vi "USBL_UA TRACKER for boat_rev2.vi"() -> ()   [LabVIEW 2017]
uses:
  <vilib>/Analysis/2dsp.llb/Decimate (single shot, DBL).vi
  <vilib>/DAQmx/read.llb/DAQmx Read (Analog 1D Wfm NChan NSamp).vi
  <vilib>/Analysis/3filter.llb/FIR Filter (DBL).vi
  <vilib>/DAQmx/create/channels.llb/DAQmx Create Channel (AI-Voltage-Basic).vi
  <vilib>/DAQmx/configure/timing.llb/DAQmx Timing (Sample Clock).vi
  <vilib>/DAQmx/miscellaneous.llb/DAQmx Fill In Error Info.vi
  <vilib>/DAQmx/create/channels.llb/DAQmx Create Channel (CO-Pulse Generation-Frequency).vi
  <vilib>/DAQmx/configure/timing.llb/DAQmx Timing (Implicit).vi
  <vilib>/Analysis/NI_AALBase.lvlib
  <vilib>/Analysis/NI_AALPro.lvlib
  <vilib>/Analysis/NI_AAL_SigProc.lvlib
  <resource>/objmgr/daqmx.rc
panel:
  out "숫자형 8":dbl=5.0
  out "Target code":dbl[](array[numeric])
  out "ThresholdMargin":dbl=10.0
  out "MovingAvrParm":dbl[](array[numeric])
  out "Coefficient_bit1":dbl[](array[numeric])
  out "Coefficient_bit0":dbl[](array[numeric])
  out "Decimation rate":i32=12
  out "Carrier signal":dbl[](array[numeric])
  out "숫자형 7":dbl=7.0
  out "숫자형 6":dbl=7.0
  out "숫자형 5":dbl=7.0
  in  "Number of pulse":i32=1000
  in  "Output terminal":tag="/Dev1/PFI12"
  in  "Frequency(Hz)":dbl=1.0 format="%.6f"
  in  "Cycle share":dbl=0.5 format="%.6f"
  in  "Counter":tag="Dev1/ctr0"
  out "Detect":bool
  in  "User number":i32=12
  out "숫자형 4":dbl=5.0
  out "숫자형 3":dbl=7.0
  out "숫자형 2":dbl=7.0
  out "숫자형":dbl=7.0
  in  "Start frequency(Hz)":dbl format="%#_6p"
  in  "Stop frequency(Hz)":dbl=4000.0 format="%#_6p"
  in  "Symbol length(sec)":dbl=0.128 format="%#_6p"
  in  "Number of sample":i32=38400
  in  "Sampling freuqncy(Hz)":dbl=192000.0 format="%#_6p"
  in  "Physical channel":tag="Dev4/ai0:7" caption="Physical Channel"
  in  "Device":tag="Dev4"
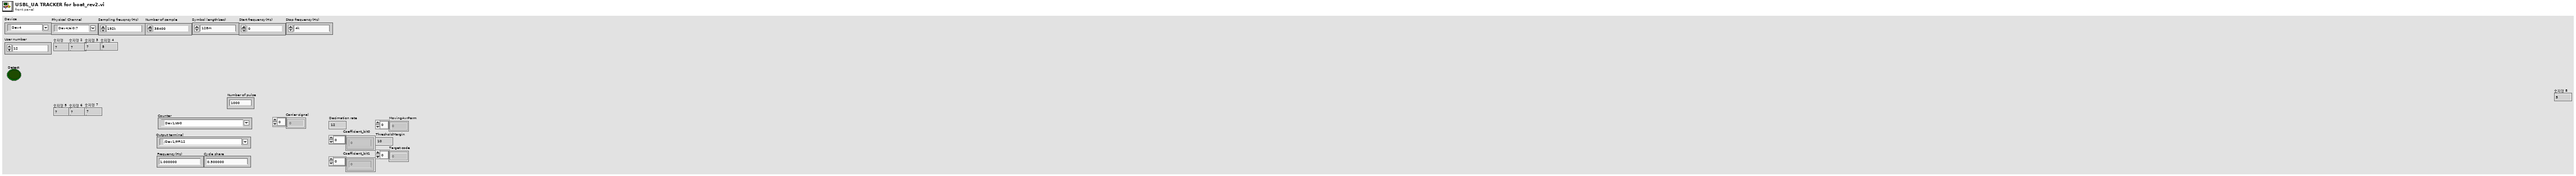
[diagram p1: front panel]
diagram:
  n1 = flat-sequence {
    tunnel: ["Number of sample"] -> w12
    tunnel: [w39] -> w11
    tunnel: ["Sampling freuqncy(Hz)"] -> w10
    tunnel: ["Physical channel"] -> w9
    tunnel: ["Device"] -> w8
    tunnel: [w35] -> w7
    tunnel: [w31] -> w6
    tunnel: [w30] -> w5
    tunnel: [w25] -> w4
    tunnel: [w21] -> w3
    tunnel: [w20] -> w2
    tunnel: [w13] -> w1
    tunnel: w12 -> [w59]
    tunnel: w11 -> [w58]
    tunnel: w10 -> [w57]
    tunnel: w9 -> [w56]
    tunnel: w8 -> [w55]
    tunnel: w7 -> [w54]
    tunnel: w6 -> [w53]
    tunnel: w5 -> [w52]
    tunnel: w4 -> [w49]
    tunnel: w3 -> [w47]
    tunnel: w2 -> [w46]
    tunnel: w1 -> [w43]
    frame #0 {
      w20 = 10.0 ("값")
      w22 = 160 ("차원 크기")
      w35 = 12 ("Divide by")
      w39 = 10123 items=["유한 샘플"=10178, "연속 샘플"=10123, "하드웨어 타이밍에 의한 단일 포인트"=12522] ("sample mode")
      # "Signal gen. (Counter)"
      # "Target code"
      # "EOF"
      # "SOF"
      # "Processing parameter"
      # "Freqeuncy 2"
      # "Freqeuncy 1"
      # "Symbol length"
      # "Moving average window size"
      # "Threshold Margin"
      # "DAQ device setting"
      # "Device"
      # "Physical channel"
      # "Sampling frequency"
      # "Sample mode"
      # "Number of samples per channel"
      n2 = To Double Precision Float(number=w35) -> (double precision float=w41:dbl)
      n3 = To Double Precision Float(number=w22) -> (double precision float=w24:dbl)
      n4 = Divide(x="Sampling freuqncy(Hz)", y=w41) -> (x/y=w29:dbl)
      n5 = Format Into String(format string="%04b" ("포맷 문자열"), "User number") -> (resulting string=w17:string)  [unwired: 2 in, 1 out]
      n6 = Reciprocal(x=w24) -> (1/x=w23:dbl)
      n7 = call "CodeConvert(SubVI).vi"("Code"=w17) -> ("Code_array"=w15:dbl[])
      n8 = Divide(x=30000.0, y="Sampling freuqncy(Hz)") -> (x/y=w33:dbl)
      n9 = Initialize Array(w23, w22) -> (w21:dbl[])
      "MovingAvrParm" <- w21
      n10 = call "ChirpSourceGen(SubVI).vi"("Frequency2(Hz)"="Stop frequency(Hz)", "Frequency1(Hz)"="Start frequency(Hz)", "Pulse length(sec)"="Symbol length(sec)", "Fs(Hz)"=w29) -> ("M.F. Tap(F2-1)"=w25:dbl[], "M.F. Tap(F1-2)"=w31:dbl[])  [unwired: 1 out]
      "Coefficient_bit0" <- w31
      "Coefficient_bit1" <- w25
      n11 = Insert Into Array(array=dbl[] [0.0, 1.0], new element #1=w15, new element #2=dbl[] [1.0, 0.0]) -> (w13:dbl[])  [unwired: 1 in]
      "Target code" <- w13
      n12 = call <vilib>:"Sine Wave.vi"("samples"="Number of sample", "amplitude"=5.0, "frequency"=w33) -> ("sine wave"=w30:dbl[])  [unwired: 2 in, 2 out]
      "Carrier signal" <- w30
      "Decimation rate" <- w35
      "ThresholdMargin" <- w20
    }
    frame #1 {
      n13 = flat-sequence {
        tunnel: w55 -> [w78]
        tunnel: [w79] -> w66
        tunnel: w56 -> [w77]
        tunnel: [w77] -> w65
        tunnel: w57 -> [w75]
        tunnel: [w75] -> w64
        tunnel: w59 -> [w74]
        tunnel: [w74] -> w63
        tunnel: w58 -> [w76]
        tunnel: [w76] -> w62
        tunnel: [w72] -> w61
        tunnel: [w73] -> w60
        tunnel: w54 -> [w73]
        tunnel: w53 -> [w72]
        tunnel: w52 -> [w71]
        tunnel: [w71] -> w51
        tunnel: [w70] -> w50
        tunnel: w49 -> [w70]
        tunnel: [w69] -> w48
        tunnel: w47 -> [w69]
        tunnel: w46 -> [w68]
        tunnel: [w68] -> w45
        tunnel: [w67] -> w44
        tunnel: w43 -> [w67]
        tunnel: w66 -> [w123]
        tunnel: w65 -> [w122]
        tunnel: w64 -> [w121]
        tunnel: w63 -> [w119]
        tunnel: w62 -> [w120]
        tunnel: w61 -> [w108]
        tunnel: w60 -> [w96]
        tunnel: w51 -> [w97]
        tunnel: w50 -> [w81]
        tunnel: w48 -> [w88]
        tunnel: w45 -> [w87]
        tunnel: w44 -> [w82]
        tunnel: [w407] -> w42
        tunnel: w42 -> [w500]
        frame #0 {
          n14 = call <vilib>:"DAQmx Reset Device.vi"("device in"=w78) -> ("error out"=w79:errorcluster)  [unwired: 1 in, 13 out]
        }
        frame #1 {
          w94 = "Proc1" ("이름(이름없음)")
          w95 = "Proc0" ("이름(이름없음)")
          w93 = dbl[][] []
          w109 = "SIG0" ("이름(이름없음)")
          w116 = waveform(dbl) {"t0"=timestamp(0 s since 1904-01-01), "dt"=1.0, "Y"=[]} ("Waveform")
          w99 = "SIG1" ("이름(이름없음)")
          # "Target code"
          # "[Post processing]  1. Queue get : Proc0, Proc1 / 2. Threshold estimation with moving average / 3. Peak and valley detection / 4. Demodulation"
          # "[Signal processing]\n1. Queue get : SIG0\n2. Data type converting : Waveform (DBL) --> Array (DBL)\n3. DDC (Digital to Digital Convering)\n  - DSB modulation : Multiply carrier signal (30kHz)\n  - Decimate : 192kHz sample rate --> 16kHz sample rate\n4. Cross-correlation with down-chirp (4k ~ 0Hz)\n5. Envelope detection (Hilbert transform) & square\n6. Queue put : Proc1"
          # "[Signal processing]\n1. Queue get : SIG0\n2. Data type converting : Waveform (DBL) --> Array (DBL)\n3. DDC (Digital to Digital Convering)\n  - DSB modulation : Multiply carrier signal (30kHz)\n  - Decimate : 192kHz sample rate --> 16kHz sample rate\n4. Cross-correlation with up-chirp (0 ~ 4kHz)\n5. Envelope detection (Hilbert transform) & square\n6. Queue put : Proc0"
          # "[Data Acquistion (ADC)]\n1. Device reset\n2. Creat channel\n3, Set sample clock\n  - Sampling frequency : 192kHz\n  - Number of sample (Chunk size) : 38400\n4. Start task\n5. Data read\n6. Queue put : SIG0, SIG1\n  - Queue data type : Waveform (DBL)"
          # "Moving average prameter based on FIR filter calculation"
          # "Coefficient for bit 1 : Down-chirp"
          # "Coefficient for bit 0 : Up-chirp"
          # "Decimation rate"
          # "Carrier signal"
          n15 = call-poly <vilib>:"DAQmx Create Virtual Channel.vi"("physical channels"=w122, "error in"=w123) -> ("task out"=w125:refnum<k21>, "error out"=w124:errorcluster)  [unwired: 7 in, 5 out]
          n16 = call-poly <vilib>:"DAQmx Timing.vi"("task/channels in"=w125, "sample mode"=w120, "samples per channel"=w119, "rate"=w121, "error in"=w124) -> ("task out"=w126:refnum<k21>, "error out"=w127:errorcluster)  [unwired: 2 in, 7 out]
          n17 = call <vilib>:"DAQmx Start Task.vi"("task/channels in"=w126, "error in"=w127) -> ("task out"=w128:refnum<k21>, "error out"=w129:errorcluster)  [unwired: 12 in]
          n18 = Build Array(w116, w116, w116, w116, w116, w116, w116, w116) -> (w98:waveform(dbl)[])
          n19 = Obtain Queue(name (unnamed)=w99, element data type=w98) -> (queue out=w118:refnum<queue>, error out=w117:errorcluster)  [unwired: 3 in, 1 out]
          n20 = Obtain Queue(name (unnamed)=w109, element data type=w98) -> (queue out=w115:refnum<queue>, error out=w114:errorcluster)  [unwired: 3 in, 1 out]
          n21 = while {
            tunnel: w128 -> [w406]
            tunnel: w129 -> [w405]
            tunnel: [w404] -> w132
            tunnel: [w403] -> w133
            tunnel: w119 -> [w402]
            tunnel: w118 -> [w401]
            tunnel: w117 -> [w400]
            tunnel: w115 -> [w399]
            tunnel: w114 -> [w398]
            i -> [w396]
            stop <- w395 stop-if-true
            n22 = call-poly <vilib>:"DAQmx Read.vi"("task/channels in"=w406, "number of samples per channel"=w402, "error in"=w405) -> ("task out"=w404:refnum<k21>, "data"=w397:waveform(dbl)[], "error out"=w403:errorcluster)  [unwired: 10 out]
            n23 = Enqueue Element(queue=w399, element=w397, error in (no error)=w398) -> ()  [unwired: 1 in, 3 out]
            n24 = Enqueue Element(queue=w401, element=w397, error in (no error)=w400) -> ()  [unwired: 1 in, 3 out]
            n25 = local read "Detect"() -> (w395:bool)
            "숫자형" <- w396
          }
          n26 = call <vilib>:"DAQmx Stop Task.vi"("task/channels in"=w132, "error in"=w133) -> ("task out"=w131:refnum<k21>, "error out"=w130:errorcluster)  [unwired: 12 out]
          n27 = call <vilib>:"DAQmx Clear Task.vi"("task in"=w131, "error in"=w130) -> ()  [unwired: 14 out]
          n28 = Obtain Queue(name (unnamed)=w95, element data type=w93) -> (queue out=w113:refnum<queue>, error out=w112:errorcluster)  [unwired: 3 in, 1 out]
          n29 = Obtain Queue(name (unnamed)=w109, element data type=w98) -> (queue out=w111:refnum<queue>, error out=w110:errorcluster)  [unwired: 3 in, 1 out]
          n30 = while {
            tunnel: w111 -> [w394]
            tunnel: w110 -> [w393]
            tunnel: w113 -> [w392]
            tunnel: w112 -> [w391]
            tunnel: [w390] -> w107
            tunnel: [w389] -> w106
            tunnel: w97 -> [w329]
            tunnel: w96 -> [w328]
            tunnel: w108 -> [w327]
            i -> [w325]
            stop <- w324 stop-if-true
            w339 = TRUE ("averaging")
            w388 = TRUE ("init/cont (init:F)")
            n31 = Dequeue Element(queue=w394, error in (no error)=w393) -> (queue out=w390:refnum<queue>, element=w330:waveform(dbl)[], error out=w389:errorcluster)  [unwired: 2 out]
            n32 = Index Array(array=w330) -> (element #1=w387:waveform(dbl), element #2=w386:waveform(dbl), element #3=w385:waveform(dbl), element #4=w384:waveform(dbl), element #5=w383:waveform(dbl), element #6=w382:waveform(dbl), element #7=w381:waveform(dbl), element #8=w380:waveform(dbl))  [unwired: 8 in]
            n33 = Unbundle By Name(w387) -> ("Y"=w379:dbl[])
            n34 = Unbundle By Name(w386) -> ("Y"=w378:dbl[])
            n35 = Unbundle By Name(w385) -> ("Y"=w377:dbl[])
            n36 = Unbundle By Name(w384) -> ("Y"=w376:dbl[])
            n37 = Unbundle By Name(w383) -> ("Y"=w375:dbl[])
            n38 = Unbundle By Name(w382) -> ("Y"=w374:dbl[])
            n39 = Unbundle By Name(w381) -> ("Y"=w373:dbl[])
            n40 = Unbundle By Name(w380) -> ("Y"=w372:dbl[])
            n41 = Multiply(x=w379, y=w329) -> (x*y=w354:dbl[])
            n42 = Multiply(x=w378, y=w329) -> (x*y=w353:dbl[])
            n43 = Multiply(x=w377, y=w329) -> (x*y=w352:dbl[])
            n44 = Multiply(x=w376, y=w329) -> (x*y=w351:dbl[])
            n45 = Multiply(x=w375, y=w329) -> (x*y=w350:dbl[])
            n46 = Multiply(x=w374, y=w329) -> (x*y=w349:dbl[])
            n47 = Multiply(x=w373, y=w329) -> (x*y=w348:dbl[])
            n48 = Multiply(x=w372, y=w329) -> (x*y=w347:dbl[])
            n49 = call-poly <vilib>:"Decimate (single shot).vi"("averaging"=w339, "decimating factor"=w328, "X"=w349) -> ("Decimated Array"=w342:dbl[])  [unwired: 7 in, 1 out]
            n50 = call-poly <vilib>:"Decimate (single shot).vi"("averaging"=w339, "decimating factor"=w328, "X"=w347) -> ("Decimated Array"=w340:dbl[])  [unwired: 7 in, 1 out]
            n51 = call-poly <vilib>:"Decimate (single shot).vi"("averaging"=w339, "decimating factor"=w328, "X"=w353) -> ("Decimated Array"=w346:dbl[])  [unwired: 7 in, 1 out]
            n52 = call-poly <vilib>:"Decimate (single shot).vi"("averaging"=w339, "decimating factor"=w328, "X"=w351) -> ("Decimated Array"=w344:dbl[])  [unwired: 7 in, 1 out]
            n53 = call-poly <vilib>:"Decimate (single shot).vi"("averaging"=w339, "decimating factor"=w328, "X"=w350) -> ("Decimated Array"=w343:dbl[])  [unwired: 7 in, 1 out]
            n54 = call-poly <vilib>:"Decimate (single shot).vi"("averaging"=w339, "decimating factor"=w328, "X"=w348) -> ("Decimated Array"=w341:dbl[])  [unwired: 7 in, 1 out]
            n55 = call-poly <vilib>:"Decimate (single shot).vi"("averaging"=w339, "decimating factor"=w328, "X"=w354) -> ("Decimated Array"=w355:dbl[])  [unwired: 7 in, 1 out]
            n56 = call-poly <vilib>:"Decimate (single shot).vi"("averaging"=w339, "decimating factor"=w328, "X"=w352) -> ("Decimated Array"=w345:dbl[])  [unwired: 7 in, 1 out]
            n57 = call-poly <vilib>:"FIR Filter.vi"("init/cont (init:F)"=w388, "FIR Coefficients"=w327, "X"=w355) -> ("Filtered X"=w371:dbl[])  [unwired: 1 in, 1 out]
            n58 = call-poly <vilib>:"FIR Filter.vi"("init/cont (init:F)"=w388, "FIR Coefficients"=w327, "X"=w346) -> ("Filtered X"=w370:dbl[])  [unwired: 1 in, 1 out]
            n59 = call-poly <vilib>:"FIR Filter.vi"("init/cont (init:F)"=w388, "FIR Coefficients"=w327, "X"=w345) -> ("Filtered X"=w369:dbl[])  [unwired: 1 in, 1 out]
            n60 = call-poly <vilib>:"FIR Filter.vi"("init/cont (init:F)"=w388, "FIR Coefficients"=w327, "X"=w344) -> ("Filtered X"=w368:dbl[])  [unwired: 1 in, 1 out]
            n61 = call-poly <vilib>:"FIR Filter.vi"("init/cont (init:F)"=w388, "FIR Coefficients"=w327, "X"=w343) -> ("Filtered X"=w367:dbl[])  [unwired: 1 in, 1 out]
            n62 = call-poly <vilib>:"FIR Filter.vi"("init/cont (init:F)"=w388, "FIR Coefficients"=w327, "X"=w342) -> ("Filtered X"=w366:dbl[])  [unwired: 1 in, 1 out]
            n63 = call-poly <vilib>:"FIR Filter.vi"("init/cont (init:F)"=w388, "FIR Coefficients"=w327, "X"=w341) -> ("Filtered X"=w365:dbl[])  [unwired: 1 in, 1 out]
            n64 = call-poly <vilib>:"FIR Filter.vi"("init/cont (init:F)"=w388, "FIR Coefficients"=w327, "X"=w340) -> ("Filtered X"=w364:dbl[])  [unwired: 1 in, 1 out]
            n65 = call "Envelope(SubVI).vi"("x"=w371) -> ("Y"=w363:dbl[])
            n66 = call "Envelope(SubVI).vi"("x"=w370) -> ("Y"=w362:dbl[])
            n67 = call "Envelope(SubVI).vi"("x"=w369) -> ("Y"=w361:dbl[])
            n68 = call "Envelope(SubVI).vi"("x"=w368) -> ("Y"=w360:dbl[])
            n69 = call "Envelope(SubVI).vi"("x"=w367) -> ("Y"=w359:dbl[])
            n70 = call "Envelope(SubVI).vi"("x"=w366) -> ("Y"=w358:dbl[])
            n71 = call "Envelope(SubVI).vi"("x"=w365) -> ("Y"=w357:dbl[])
            n72 = call "Envelope(SubVI).vi"("x"=w364) -> ("Y"=w356:dbl[])
            n73 = Square(x=w363) -> (x^2=w338:dbl[])
            n74 = Square(x=w362) -> (x^2=w337:dbl[])
            n75 = Square(x=w361) -> (x^2=w336:dbl[])
            n76 = Square(x=w360) -> (x^2=w335:dbl[])
            n77 = Square(x=w359) -> (x^2=w334:dbl[])
            n78 = Square(x=w358) -> (x^2=w333:dbl[])
            n79 = Square(x=w357) -> (x^2=w332:dbl[])
            n80 = Square(x=w356) -> (x^2=w331:dbl[])
            n81 = local read "Detect"() -> (w324:bool)
            n82 = Build Array(w338, w337, w336, w335, w334, w333, w332, w331) -> (w326:dbl[][])
            n83 = Enqueue Element(queue=w392, element=w326, error in (no error)=w391) -> ()  [unwired: 1 in, 3 out]
            "숫자형 2" <- w325
          }
          n84 = Release Queue(queue=w107, error in (no error)=w106) -> ()  [unwired: 1 in, 3 out]
          n85 = Obtain Queue(name (unnamed)=w94, element data type=w93) -> (queue out=w105:refnum<queue>, error out=w104:errorcluster)  [unwired: 3 in, 1 out]
          n86 = Obtain Queue(name (unnamed)=w99, element data type=w98) -> (queue out=w103:refnum<queue>, error out=w102:errorcluster)  [unwired: 3 in, 1 out]
          n87 = while {
            tunnel: w103 -> [w323]
            tunnel: w102 -> [w322]
            tunnel: w105 -> [w321]
            tunnel: w104 -> [w320]
            tunnel: [w319] -> w101
            tunnel: [w318] -> w100
            tunnel: w97 -> [w258]
            tunnel: w96 -> [w257]
            tunnel: w81 -> [w256]
            i -> [w254]
            stop <- w253 stop-if-true
            w268 = TRUE ("averaging")
            w317 = TRUE ("init/cont (init:F)")
            n88 = Dequeue Element(queue=w323, error in (no error)=w322) -> (queue out=w319:refnum<queue>, element=w259:waveform(dbl)[], error out=w318:errorcluster)  [unwired: 2 out]
            n89 = Index Array(array=w259) -> (element #1=w316:waveform(dbl), element #2=w315:waveform(dbl), element #3=w314:waveform(dbl), element #4=w313:waveform(dbl), element #5=w312:waveform(dbl), element #6=w311:waveform(dbl), element #7=w310:waveform(dbl), element #8=w309:waveform(dbl))  [unwired: 8 in]
            n90 = Unbundle By Name(w316) -> ("Y"=w308:dbl[])
            n91 = Unbundle By Name(w315) -> ("Y"=w307:dbl[])
            n92 = Unbundle By Name(w314) -> ("Y"=w306:dbl[])
            n93 = Unbundle By Name(w313) -> ("Y"=w305:dbl[])
            n94 = Unbundle By Name(w312) -> ("Y"=w304:dbl[])
            n95 = Unbundle By Name(w311) -> ("Y"=w303:dbl[])
            n96 = Unbundle By Name(w310) -> ("Y"=w302:dbl[])
            n97 = Unbundle By Name(w309) -> ("Y"=w301:dbl[])
            n98 = Multiply(x=w308, y=w258) -> (x*y=w283:dbl[])
            n99 = Multiply(x=w307, y=w258) -> (x*y=w282:dbl[])
            n100 = Multiply(x=w306, y=w258) -> (x*y=w281:dbl[])
            n101 = Multiply(x=w305, y=w258) -> (x*y=w280:dbl[])
            n102 = Multiply(x=w304, y=w258) -> (x*y=w279:dbl[])
            n103 = Multiply(x=w303, y=w258) -> (x*y=w278:dbl[])
            n104 = Multiply(x=w302, y=w258) -> (x*y=w277:dbl[])
            n105 = Multiply(x=w301, y=w258) -> (x*y=w276:dbl[])
            n106 = call-poly <vilib>:"Decimate (single shot).vi"("averaging"=w268, "decimating factor"=w257, "X"=w278) -> ("Decimated Array"=w271:dbl[])  [unwired: 7 in, 1 out]
            n107 = call-poly <vilib>:"Decimate (single shot).vi"("averaging"=w268, "decimating factor"=w257, "X"=w276) -> ("Decimated Array"=w269:dbl[])  [unwired: 7 in, 1 out]
            n108 = call-poly <vilib>:"Decimate (single shot).vi"("averaging"=w268, "decimating factor"=w257, "X"=w282) -> ("Decimated Array"=w275:dbl[])  [unwired: 7 in, 1 out]
            n109 = call-poly <vilib>:"Decimate (single shot).vi"("averaging"=w268, "decimating factor"=w257, "X"=w280) -> ("Decimated Array"=w273:dbl[])  [unwired: 7 in, 1 out]
            n110 = call-poly <vilib>:"Decimate (single shot).vi"("averaging"=w268, "decimating factor"=w257, "X"=w279) -> ("Decimated Array"=w272:dbl[])  [unwired: 7 in, 1 out]
            n111 = call-poly <vilib>:"Decimate (single shot).vi"("averaging"=w268, "decimating factor"=w257, "X"=w277) -> ("Decimated Array"=w270:dbl[])  [unwired: 7 in, 1 out]
            n112 = call-poly <vilib>:"Decimate (single shot).vi"("averaging"=w268, "decimating factor"=w257, "X"=w283) -> ("Decimated Array"=w284:dbl[])  [unwired: 7 in, 1 out]
            n113 = call-poly <vilib>:"Decimate (single shot).vi"("averaging"=w268, "decimating factor"=w257, "X"=w281) -> ("Decimated Array"=w274:dbl[])  [unwired: 7 in, 1 out]
            n114 = call-poly <vilib>:"FIR Filter.vi"("init/cont (init:F)"=w317, "FIR Coefficients"=w256, "X"=w284) -> ("Filtered X"=w300:dbl[])  [unwired: 1 in, 1 out]
            n115 = call-poly <vilib>:"FIR Filter.vi"("init/cont (init:F)"=w317, "FIR Coefficients"=w256, "X"=w275) -> ("Filtered X"=w299:dbl[])  [unwired: 1 in, 1 out]
            n116 = call-poly <vilib>:"FIR Filter.vi"("init/cont (init:F)"=w317, "FIR Coefficients"=w256, "X"=w274) -> ("Filtered X"=w298:dbl[])  [unwired: 1 in, 1 out]
            n117 = call-poly <vilib>:"FIR Filter.vi"("init/cont (init:F)"=w317, "FIR Coefficients"=w256, "X"=w273) -> ("Filtered X"=w297:dbl[])  [unwired: 1 in, 1 out]
            n118 = call-poly <vilib>:"FIR Filter.vi"("init/cont (init:F)"=w317, "FIR Coefficients"=w256, "X"=w272) -> ("Filtered X"=w296:dbl[])  [unwired: 1 in, 1 out]
            n119 = call-poly <vilib>:"FIR Filter.vi"("init/cont (init:F)"=w317, "FIR Coefficients"=w256, "X"=w271) -> ("Filtered X"=w295:dbl[])  [unwired: 1 in, 1 out]
            n120 = call-poly <vilib>:"FIR Filter.vi"("init/cont (init:F)"=w317, "FIR Coefficients"=w256, "X"=w270) -> ("Filtered X"=w294:dbl[])  [unwired: 1 in, 1 out]
            n121 = call-poly <vilib>:"FIR Filter.vi"("init/cont (init:F)"=w317, "FIR Coefficients"=w256, "X"=w269) -> ("Filtered X"=w293:dbl[])  [unwired: 1 in, 1 out]
            n122 = call "Envelope(SubVI).vi"("x"=w300) -> ("Y"=w292:dbl[])
            n123 = call "Envelope(SubVI).vi"("x"=w299) -> ("Y"=w291:dbl[])
            n124 = call "Envelope(SubVI).vi"("x"=w298) -> ("Y"=w290:dbl[])
            n125 = call "Envelope(SubVI).vi"("x"=w297) -> ("Y"=w289:dbl[])
            n126 = call "Envelope(SubVI).vi"("x"=w296) -> ("Y"=w288:dbl[])
            n127 = call "Envelope(SubVI).vi"("x"=w295) -> ("Y"=w287:dbl[])
            n128 = call "Envelope(SubVI).vi"("x"=w294) -> ("Y"=w286:dbl[])
            n129 = call "Envelope(SubVI).vi"("x"=w293) -> ("Y"=w285:dbl[])
            n130 = Square(x=w292) -> (x^2=w267:dbl[])
            n131 = Square(x=w291) -> (x^2=w266:dbl[])
            n132 = Square(x=w290) -> (x^2=w265:dbl[])
            n133 = Square(x=w289) -> (x^2=w264:dbl[])
            n134 = Square(x=w288) -> (x^2=w263:dbl[])
            n135 = Square(x=w287) -> (x^2=w262:dbl[])
            n136 = Square(x=w286) -> (x^2=w261:dbl[])
            n137 = Square(x=w285) -> (x^2=w260:dbl[])
            n138 = local read "Detect"() -> (w253:bool)
            n139 = Build Array(w267, w266, w265, w264, w263, w262, w261, w260) -> (w255:dbl[][])
            n140 = Enqueue Element(queue=w321, element=w255, error in (no error)=w320) -> ()  [unwired: 1 in, 3 out]
            "숫자형 3" <- w254
          }
          n141 = Release Queue(queue=w101, error in (no error)=w100) -> ()  [unwired: 1 in, 3 out]
          n142 = Obtain Queue(name (unnamed)=w95, element data type=w93) -> (queue out=w92:refnum<queue>, error out=w91:errorcluster)  [unwired: 3 in, 1 out]
          n143 = Obtain Queue(name (unnamed)=w94, element data type=w93) -> (queue out=w90:refnum<queue>, error out=w89:errorcluster)  [unwired: 3 in, 1 out]
          n144 = while {
            tunnel: w92 -> [w252]
            tunnel: w91 -> [w251]
            tunnel: w90 -> [w250]
            tunnel: w89 -> [w249]
            tunnel: w88 -> [w247]
            tunnel: w87 -> [w211]
            tunnel: [w191] -> w86
            tunnel: [w190] -> w85
            tunnel: [w189] -> w84
            tunnel: [w188] -> w83
            tunnel: w82 -> [w187]
            shift-right: [w136] -> _
            shift-left: dbl[][] [[-1.0, -1.0, -1.0, -1.0, -1.0, -1.0, -1.0, -1.0], [-1.0, -1.0, -1.0, -1.0, -1.0, -1.0, -1.0, -1.0]] -> [w141]
            i -> [w140]
            stop <- w176 stop-if-true
            w236 = enum32{"Peaks", "Valleys"}."Valleys" ("peaks/valleys")
            w237 = enum32{"Peaks", "Valleys"}."Peaks" ("peaks/valleys")
            w235 = 5 ("width")
            w246 = TRUE ("init/cont (init:F)")
            n145 = Dequeue Element(queue=w252, error in (no error)=w251) -> (queue out=w191:refnum<queue>, element=w193:dbl[][], error out=w190:errorcluster)  [unwired: 2 out]
            n146 = Dequeue Element(queue=w250, error in (no error)=w249) -> (queue out=w189:refnum<queue>, element=w192:dbl[][], error out=w188:errorcluster)  [unwired: 2 out]
            n147 = Subtract(x=w193, y=w192) -> (x-y=w248:dbl[][])
            n148 = Index Array(array=w248) -> (element #1=w234:dbl[], element #2=w233:dbl[], element #3=w232:dbl[], element #4=w231:dbl[], element #5=w230:dbl[], element #6=w229:dbl[], element #7=w228:dbl[], element #8=w196:dbl[])  [unwired: 16 in]
            n149 = call-poly <vilib>:"FIR Filter.vi"("init/cont (init:F)"=w246, "FIR Coefficients"=w247, "X"=w234) -> ("Filtered X"=w245:dbl[])  [unwired: 1 in, 1 out]
            n150 = call-poly <vilib>:"FIR Filter.vi"("init/cont (init:F)"=w246, "FIR Coefficients"=w247, "X"=w233) -> ("Filtered X"=w244:dbl[])  [unwired: 1 in, 1 out]
            n151 = call-poly <vilib>:"FIR Filter.vi"("init/cont (init:F)"=w246, "FIR Coefficients"=w247, "X"=w232) -> ("Filtered X"=w243:dbl[])  [unwired: 1 in, 1 out]
            n152 = call-poly <vilib>:"FIR Filter.vi"("init/cont (init:F)"=w246, "FIR Coefficients"=w247, "X"=w231) -> ("Filtered X"=w242:dbl[])  [unwired: 1 in, 1 out]
            n153 = call-poly <vilib>:"FIR Filter.vi"("init/cont (init:F)"=w246, "FIR Coefficients"=w247, "X"=w230) -> ("Filtered X"=w241:dbl[])  [unwired: 1 in, 1 out]
            n154 = call-poly <vilib>:"FIR Filter.vi"("init/cont (init:F)"=w246, "FIR Coefficients"=w247, "X"=w229) -> ("Filtered X"=w240:dbl[])  [unwired: 1 in, 1 out]
            n155 = call-poly <vilib>:"FIR Filter.vi"("init/cont (init:F)"=w246, "FIR Coefficients"=w247, "X"=w228) -> ("Filtered X"=w239:dbl[])  [unwired: 1 in, 1 out]
            n156 = call-poly <vilib>:"FIR Filter.vi"("init/cont (init:F)"=w246, "FIR Coefficients"=w247, "X"=w196) -> ("Filtered X"=w238:dbl[])  [unwired: 1 in, 1 out]
            n157 = Array Max & Min(array=w245) -> (max value=w227:dbl, min value=w226:dbl)  [unwired: 2 out]
            n158 = Array Max & Min(array=w244) -> (max value=w225:dbl, min value=w224:dbl)  [unwired: 2 out]
            n159 = Array Max & Min(array=w243) -> (max value=w223:dbl, min value=w222:dbl)  [unwired: 2 out]
            n160 = Array Max & Min(array=w242) -> (max value=w221:dbl, min value=w220:dbl)  [unwired: 2 out]
            n161 = Array Max & Min(array=w241) -> (max value=w219:dbl, min value=w218:dbl)  [unwired: 2 out]
            n162 = Array Max & Min(array=w240) -> (max value=w217:dbl, min value=w216:dbl)  [unwired: 2 out]
            n163 = Array Max & Min(array=w239) -> (max value=w215:dbl, min value=w214:dbl)  [unwired: 2 out]
            n164 = Array Max & Min(array=w238) -> (max value=w213:dbl, min value=w212:dbl)  [unwired: 2 out]
            n165 = call "ThresholdEstimation(SubVI).vi"("Margin"=w211, "최소값"=w224, "최대값"=w225) -> ("N.Th"=w198:dbl, "P.Th"=w209:dbl)
            n166 = call "ThresholdEstimation(SubVI).vi"("Margin"=w211, "최소값"=w222, "최대값"=w223) -> ("N.Th"=w199:dbl, "P.Th"=w208:dbl)
            n167 = call "ThresholdEstimation(SubVI).vi"("Margin"=w211, "최소값"=w220, "최대값"=w221) -> ("N.Th"=w200:dbl, "P.Th"=w207:dbl)
            n168 = call "ThresholdEstimation(SubVI).vi"("Margin"=w211, "최소값"=w218, "최대값"=w219) -> ("N.Th"=w201:dbl, "P.Th"=w206:dbl)
            n169 = call "ThresholdEstimation(SubVI).vi"("Margin"=w211, "최소값"=w226, "최대값"=w227) -> ("N.Th"=w197:dbl, "P.Th"=w210:dbl)
            n170 = call "ThresholdEstimation(SubVI).vi"("Margin"=w211, "최소값"=w216, "최대값"=w217) -> ("N.Th"=w202:dbl, "P.Th"=w205:dbl)
            n171 = call "ThresholdEstimation(SubVI).vi"("Margin"=w211, "최소값"=w214, "최대값"=w215) -> ("N.Th"=w203:dbl, "P.Th"=w204:dbl)
            n172 = call "ThresholdEstimation(SubVI).vi"("Margin"=w211, "최소값"=w212, "최대값"=w213) -> ("N.Th"=w195:dbl, "P.Th"=w194:dbl)
            n173 = call <vilib>:"Peak Detector.vi"("peaks/valleys"=w237, "width"=w235, "threshold"=w210, "X"=w234) -> ("Locations"=w173:dbl[], "# found"=w175:i32)  [unwired: 3 in, 3 out]
            n174 = call <vilib>:"Peak Detector.vi"("peaks/valleys"=w237, "width"=w235, "threshold"=w209, "X"=w233) -> ("Locations"=w169:dbl[], "# found"=w171:i32)  [unwired: 3 in, 3 out]
            n175 = call <vilib>:"Peak Detector.vi"("peaks/valleys"=w237, "width"=w235, "threshold"=w208, "X"=w232) -> ("Locations"=w165:dbl[], "# found"=w167:i32)  [unwired: 3 in, 3 out]
            n176 = call <vilib>:"Peak Detector.vi"("peaks/valleys"=w237, "width"=w235, "threshold"=w207, "X"=w231) -> ("Locations"=w161:dbl[], "# found"=w163:i32)  [unwired: 3 in, 3 out]
            n177 = call <vilib>:"Peak Detector.vi"("peaks/valleys"=w237, "width"=w235, "threshold"=w206, "X"=w230) -> ("Locations"=w157:dbl[], "# found"=w159:i32)  [unwired: 3 in, 3 out]
            n178 = call <vilib>:"Peak Detector.vi"("peaks/valleys"=w237, "width"=w235, "threshold"=w205, "X"=w229) -> ("Locations"=w153:dbl[], "# found"=w155:i32)  [unwired: 3 in, 3 out]
            n179 = call <vilib>:"Peak Detector.vi"("peaks/valleys"=w237, "width"=w235, "threshold"=w204, "X"=w228) -> ("Locations"=w149:dbl[], "# found"=w151:i32)  [unwired: 3 in, 3 out]
            n180 = call <vilib>:"Peak Detector.vi"("peaks/valleys"=w237, "width"=w235, "threshold"=w194, "X"=w196) -> ("Locations"=w145:dbl[], "# found"=w147:i32)  [unwired: 3 in, 3 out]
            n181 = call <vilib>:"Peak Detector.vi"("peaks/valleys"=w236, "width"=w235, "threshold"=w197, "X"=w234) -> ("Locations"=w172:dbl[], "# found"=w174:i32)  [unwired: 3 in, 3 out]
            n182 = call <vilib>:"Peak Detector.vi"("peaks/valleys"=w236, "width"=w235, "threshold"=w198, "X"=w233) -> ("Locations"=w168:dbl[], "# found"=w170:i32)  [unwired: 3 in, 3 out]
            n183 = call <vilib>:"Peak Detector.vi"("peaks/valleys"=w236, "width"=w235, "threshold"=w199, "X"=w232) -> ("Locations"=w164:dbl[], "# found"=w166:i32)  [unwired: 3 in, 3 out]
            n184 = call <vilib>:"Peak Detector.vi"("peaks/valleys"=w236, "width"=w235, "threshold"=w200, "X"=w231) -> ("Locations"=w160:dbl[], "# found"=w162:i32)  [unwired: 3 in, 3 out]
            n185 = call <vilib>:"Peak Detector.vi"("peaks/valleys"=w236, "width"=w235, "threshold"=w201, "X"=w230) -> ("Locations"=w156:dbl[], "# found"=w158:i32)  [unwired: 3 in, 3 out]
            n186 = call <vilib>:"Peak Detector.vi"("peaks/valleys"=w236, "width"=w235, "threshold"=w202, "X"=w229) -> ("Locations"=w152:dbl[], "# found"=w154:i32)  [unwired: 3 in, 3 out]
            n187 = call <vilib>:"Peak Detector.vi"("peaks/valleys"=w236, "width"=w235, "threshold"=w203, "X"=w228) -> ("Locations"=w148:dbl[], "# found"=w150:i32)  [unwired: 3 in, 3 out]
            n188 = call <vilib>:"Peak Detector.vi"("peaks/valleys"=w236, "width"=w235, "threshold"=w195, "X"=w196) -> ("Locations"=w144:dbl[], "# found"=w146:i32)  [unwired: 3 in, 3 out]
            n189 = local read "Number of sample"() -> (w139:i32)
            n190 = Divide(x=w139, y=12) -> (x/y=w137:dbl)
            n191 = call "Decision2(SubVI).vi"("L_ind0"=w175, "number of sample"=w137, "L_ind1"=w174, "Peak_ind0"=w173, "index"=w140, "Peak_ind1"=w172) -> ("L_sum"=w134:i32, "Bits"=w143:dbl[], "Position"=w142:dbl[])
            n192 = call "Decision2(SubVI).vi"("L_ind0"=w171, "L_ind1"=w170, "Peak_ind0"=w169, "Peak_ind1"=w168) -> ()  [unwired: 2 in, 3 out]
            n193 = call "Decision2(SubVI).vi"("L_ind0"=w167, "L_ind1"=w166, "Peak_ind0"=w165, "Peak_ind1"=w164) -> ()  [unwired: 2 in, 3 out]
            n194 = call "Decision2(SubVI).vi"("L_ind0"=w163, "L_ind1"=w162, "Peak_ind0"=w161, "Peak_ind1"=w160) -> ()  [unwired: 2 in, 3 out]
            n195 = call "Decision2(SubVI).vi"("L_ind0"=w159, "L_ind1"=w158, "Peak_ind0"=w157, "Peak_ind1"=w156) -> ()  [unwired: 2 in, 3 out]
            n196 = call "Decision2(SubVI).vi"("L_ind0"=w155, "L_ind1"=w154, "Peak_ind0"=w153, "Peak_ind1"=w152) -> ()  [unwired: 2 in, 3 out]
            n197 = call "Decision2(SubVI).vi"("L_ind0"=w151, "L_ind1"=w150, "Peak_ind0"=w149, "Peak_ind1"=w148) -> ()  [unwired: 2 in, 3 out]
            n198 = call "Decision2(SubVI).vi"("L_ind0"=w147, "L_ind1"=w146, "Peak_ind0"=w145, "Peak_ind1"=w144) -> ()  [unwired: 2 in, 3 out]
            n199 = call "TImeThresholdLogic(SubVI).vi"("Position"=w142, "Bits"=w143, "Buffer"=w141) -> ("Data"=w136:dbl[][])  [unwired: 1 in]
            n200 = Index Array(array=w136) -> (element=w135:dbl[])  [unwired: 2 in]
            n201 = call "CodeDetection(SubVI).vi"("Code"=w187, "Buff"=w135, "L_sum"=w134) -> ("detect"=w186:bool)
            n202 = call "CodeDetection(SubVI).vi"("Code"=w187) -> ("detect"=w185:bool)  [unwired: 2 in]
            n203 = call "CodeDetection(SubVI).vi"("Code"=w187) -> ("detect"=w184:bool)  [unwired: 2 in]
            n204 = call "CodeDetection(SubVI).vi"("Code"=w187) -> ("detect"=w183:bool)  [unwired: 2 in]
            n205 = call "CodeDetection(SubVI).vi"("Code"=w187) -> ("detect"=w182:bool)  [unwired: 2 in]
            n206 = call "CodeDetection(SubVI).vi"("Code"=w187) -> ("detect"=w181:bool)  [unwired: 2 in]
            n207 = call "CodeDetection(SubVI).vi"("Code"=w187) -> ("detect"=w180:bool)  [unwired: 2 in]
            n208 = call "CodeDetection(SubVI).vi"("Code"=w187) -> ("detect"=w179:bool)  [unwired: 2 in]
            n209 = Build Array(w186, w185, w184, w183, w182, w181, w180, w179) -> (w178:bool[])
            n210 = Boolean Array To Number(Boolean array=w178) -> (number=w177:u32)
            n211 = Greater Than 0?(x=w177) -> (x > 0?=w176:bool)
            "Detect" <- w176
            "숫자형 4" <- w140
          }
          n212 = Release Queue(queue=w86, error in (no error)=w85) -> ()  [unwired: 1 in, 3 out]
          n213 = Release Queue(queue=w84, error in (no error)=w83) -> ()  [unwired: 1 in, 3 out]
        }
        frame #2 {
          n214 = local read "Device"() -> (w408:tag)
          n215 = call <vilib>:"DAQmx Reset Device.vi"("device in"=w408) -> ("error out"=w407:errorcluster)  [unwired: 1 in, 13 out]
        }
        frame #3 {
          w413 = dbl[] [-1.0, -1.0, -1.0, -1.0, -1.0, -1.0, -1.0, -1.0]
          w427 = dbl[][] []
          w443 = waveform(dbl) {"t0"=timestamp(0 s since 1904-01-01), "dt"=1.0, "Y"=[]} ("Waveform")
          w416 = "Proc1" ("이름(이름없음)")
          w415 = "Proc0" ("이름(이름없음)")
          w414 = dbl[][] []
          w466 = "SIG0" ("이름(이름없음)")
          w473 = waveform(dbl) {"t0"=timestamp(0 s since 1904-01-01), "dt"=1.0, "Y"=[]} ("Waveform")
          w457 = "SIG1" ("이름(이름없음)")
          w489 = 10123 items=["유한 샘플"=10178, "연속 샘플"=10123, "하드웨어 타이밍에 의한 단일 포인트"=12522] ("sample mode")
          w493 = 10178 items=["유한 샘플"=10178, "연속 샘플"=10123, "하드웨어 타이밍에 의한 단일 포인트"=12522] ("sample mode")
          # "[Post processing]  1. Queue get : Proc0, Proc1 / 2. Threshold estimation with moving average / 3. Peak and valley detection / 4. Demodulation"
          # "[Rx.time]\nTravel time (1km) : 670ms * 2\nDown-link : 210ms\nUp-link : 1024ms\nTotal : Rx.time > 2574ms"
          # "Local variable"
          # "Queue clear"
          # "[Data Acquistion (ADC)]"
          # "Signal generation (Counter) / delaty time : 200ms"
          # "[Signal processing]\n1. Queue get : SIG0\n2. Data type converting : Waveform (DBL) --> Array (DBL)\n3. DDC (Digital to Digital Convering)\n  - DSB modulation : Multiply carrier signal (30kHz)\n  - Decimate : 192kHz sample rate --> 16kHz sample rate\n4. Cross-correlation with down-chirp (4k ~ 0Hz)\n5. Envelope detection (Hilbert transform) & square\n6. Queue put : Proc1"
          # "[Signal processing]\n1. Queue get : SIG0\n2. Data type converting : Waveform (DBL) --> Array (DBL)\n3. DDC (Digital to Digital Convering)\n  - DSB modulation : Multiply carrier signal (30kHz)\n  - Decimate : 192kHz sample rate --> 16kHz sample rate\n4. Cross-correlation with up-chirp (0 ~ 4kHz)\n5. Envelope detection (Hilbert transform) & square\n6. Queue put : Proc0"
          # "[Data Acquistion (ADC)]\n1. Device reset\n2. Creat channel\n3, Set sample clock\n  - Sampling frequency : 192kHz\n  - Number of sample (Chunk size) : 38400\n4. Start task\n5. Data read\n6. Queue put : SIG0, SIG1\n  - Queue data type : Waveform (DBL)"
          n216 = local read "Number of pulse"() -> (w494:i32)
          n217 = local read "Output terminal"() -> (w497:tag)
          n218 = local read "Sampling freuqncy(Hz)"() -> (w425:dbl)
          n219 = local read "Physical channel"() -> (w491:tag)
          n220 = local read "Frequency(Hz)"() -> (w502:dbl)
          n221 = Build Array(w443, w443, w443, w443, w443, w443, w443, w443) -> (w442:waveform(dbl)[])
          n222 = local read "Cycle share"() -> (w501:dbl)
          n223 = local read "Number of sample"() -> (w424:i32)
          n224 = local read "Counter"() -> (w503:tag)
          n225 = Obtain Queue(name (unnamed)="SIG1" ("이름(이름없음)"), element data type=w442) -> (queue out=w439:refnum<queue>, error out=w438:errorcluster)  [unwired: 3 in, 1 out]
          n226 = Obtain Queue(name (unnamed)="Proc1" ("이름(이름없음)"), element data type=w427) -> (queue out=w431:refnum<queue>, error out=w430:errorcluster)  [unwired: 3 in, 1 out]
          n227 = Obtain Queue(name (unnamed)="SIG0" ("이름(이름없음)"), element data type=w442) -> (queue out=w449:refnum<queue>, error out=w448:errorcluster)  [unwired: 3 in, 1 out]
          n228 = Obtain Queue(name (unnamed)="Proc0" ("이름(이름없음)"), element data type=w427) -> (queue out=w437:refnum<queue>, error out=w436:errorcluster)  [unwired: 3 in, 1 out]
          n229 = call-poly <vilib>:"DAQmx Create Virtual Channel.vi"("frequency"=w502, "duty cycle"=w501, "counter"=w503, "error in"=w500) -> ("task out"=w499:refnum<k21>, "error out"=w498:errorcluster)  [unwired: 10 in]
          n230 = call-poly <vilib>:"DAQmx Create Virtual Channel.vi"("physical channels"=w491) -> ("task out"=w490:refnum<k21>, "error out"=w492:errorcluster)  [unwired: 8 in, 5 out]
          n231 = Flush Queue(queue=w449, error in (no error)=w448) -> (queue out=w447:refnum<queue>, error out=w446:errorcluster)  [unwired: 1 out]
          n232 = Flush Queue(queue=w439, error in (no error)=w438) -> (queue out=w441:refnum<queue>, error out=w440:errorcluster)  [unwired: 1 out]
          n233 = Flush Queue(queue=w437, error in (no error)=w436) -> (queue out=w435:refnum<queue>, error out=w434:errorcluster)  [unwired: 1 out]
          n234 = Flush Queue(queue=w431, error in (no error)=w430) -> (queue out=w433:refnum<queue>, error out=w432:errorcluster)  [unwired: 1 out]
          n235 = property class="DAQmx 채널"(reference=w499, error in=w498, "CO.Pulse.Term"=w497) -> (reference out=w496:refnum<k21>, error out=w495:errorcluster)
          n236 = Release Queue(queue=w447, error in (no error)=w446) -> ()  [unwired: 1 in, 3 out]
          n237 = Release Queue(queue=w441, error in (no error)=w440) -> ()  [unwired: 1 in, 3 out]
          n238 = Release Queue(queue=w435, error in (no error)=w434) -> ()  [unwired: 1 in, 3 out]
          n239 = Release Queue(queue=w433, error in (no error)=w432) -> ()  [unwired: 1 in, 3 out]
          n240 = call-poly <vilib>:"DAQmx Timing.vi"("task/channels in"=w490, "sample mode"=w489, "samples per channel"=w424, "rate"=w425, "error in"=w492) -> ("task out"=w488:refnum<k21>, "error out"=w487:errorcluster)  [unwired: 2 in, 7 out]
          n241 = call-poly <vilib>:"DAQmx Timing.vi"("task/channels in"=w496, "sample mode"=w493, "samples per channel"=w494, "error in"=w495) -> ("task out"=w486:refnum<k21>, "error out"=w485:errorcluster)  [unwired: 10 in]
          n242 = flat-sequence {
            tunnel: w488 -> [w800]
            tunnel: w487 -> [w799]
            tunnel: w486 -> [w798]
            tunnel: w485 -> [w797]
            tunnel: [w798] -> w484
            tunnel: [w797] -> w483
            tunnel: [w796] -> w455
            tunnel: [w795] -> w454
            frame #0 {
              n243 = call <vilib>:"DAQmx Start Task.vi"("task/channels in"=w800, "error in"=w799) -> ("task out"=w796:refnum<k21>, "error out"=w795:errorcluster)  [unwired: 12 in]
            }
          }
          n244 = for {
            N: 2 -> [_]
            tunnel: w484 -> [w793]
            tunnel: [w788] -> w481
            tunnel: w483 -> [w794]
            tunnel: [w787] -> w480
            n245 = call <vilib>:"DAQmx Start Task.vi"("task/channels in"=w793, "error in"=w794) -> ("task out"=w792:refnum<k21>, "error out"=w791:errorcluster)  [unwired: 12 in]
            n246 = call <vilib>:"DAQmx Is Task Done.vi"("task/channels in"=w792, "error in"=w791) -> ("task out"=w790:refnum<k21>, "error out"=w789:errorcluster)  [unwired: 11 in, 1 out]
            n247 = Wait (ms)(milliseconds to wait=u32 200 ("대기 시간 (ms)")) -> ()  [unwired: 1 out]
            n248 = call <vilib>:"DAQmx Stop Task.vi"("task/channels in"=w790, "error in"=w789) -> ("task out"=w788:refnum<k21>, "error out"=w787:errorcluster)  [unwired: 12 in]
          }
          n249 = Multiply(x=3.0, y=w425) -> (x*y=w423:dbl)
          n250 = To Double Precision Float(number=w424) -> (double precision float=w422:dbl)
          n251 = Divide(x=w423, y=w422) -> (x/y=w421:dbl)
          n252 = To Long Integer(number=w421) -> (32bit integer=w409:i32)
          n253 = call <vilib>:"DAQmx Clear Task.vi"("task in"=w481, "error in"=w480) -> ()  [unwired: 13 in, 1 out]
          n254 = Build Array(w473, w473, w473, w473, w473, w473, w473, w473) -> (w456:waveform(dbl)[])
          n255 = Obtain Queue(name (unnamed)=w457, element data type=w456) -> (queue out=w475:refnum<queue>, error out=w474:errorcluster)  [unwired: 3 in, 1 out]
          n256 = Obtain Queue(name (unnamed)=w466, element data type=w456) -> (queue out=w472:refnum<queue>, error out=w471:errorcluster)  [unwired: 3 in, 1 out]
          n257 = for {
            N: w409 -> [_]
            tunnel: w455 -> [w785]
            tunnel: w454 -> [w784]
            tunnel: [w783] -> w478
            tunnel: [w782] -> w479
            tunnel: w424 -> [w781]
            tunnel: w475 -> [w780]
            tunnel: w474 -> [w779]
            tunnel: w472 -> [w778]
            tunnel: w471 -> [w777]
            i -> [w775]
            n258 = call-poly <vilib>:"DAQmx Read.vi"("task/channels in"=w785, "number of samples per channel"=w781, "error in"=w784) -> ("task out"=w783:refnum<k21>, "data"=w776:waveform(dbl)[], "error out"=w782:errorcluster)  [unwired: 10 out]
            n259 = Enqueue Element(queue=w778, element=w776, error in (no error)=w777) -> ()  [unwired: 1 in, 3 out]
            n260 = Enqueue Element(queue=w780, element=w776, error in (no error)=w779) -> ()  [unwired: 1 in, 3 out]
            "숫자형 5" <- w775
          }
          n261 = local read "Coefficient_bit1"() -> (w450:dbl[])
          n262 = local read "ThresholdMargin"() -> (w410:dbl)
          n263 = local read "MovingAvrParm"() -> (w411:dbl[])
          n264 = local read "Decimation rate"() -> (w452:i32)
          n265 = local read "Coefficient_bit0"() -> (w451:dbl[])
          n266 = local read "Carrier signal"() -> (w453:dbl[])
          n267 = local read "Target code"() -> (w412:dbl[])
          n268 = call <vilib>:"DAQmx Stop Task.vi"("task/channels in"=w478, "error in"=w479) -> ("task out"=w477:refnum<k21>, "error out"=w476:errorcluster)  [unwired: 12 out]
          n269 = call <vilib>:"DAQmx Clear Task.vi"("task in"=w477, "error in"=w476) -> ()  [unwired: 14 out]
          n270 = Obtain Queue(name (unnamed)=w415, element data type=w414) -> (queue out=w470:refnum<queue>, error out=w469:errorcluster)  [unwired: 3 in, 1 out]
          n271 = Obtain Queue(name (unnamed)=w466, element data type=w456) -> (queue out=w468:refnum<queue>, error out=w467:errorcluster)  [unwired: 3 in, 1 out]
          n272 = for {
            N: w409 -> [_]
            tunnel: w468 -> [w774]
            tunnel: w467 -> [w773]
            tunnel: w470 -> [w772]
            tunnel: w469 -> [w771]
            tunnel: [w770] -> w465
            tunnel: [w769] -> w464
            tunnel: w453 -> [w709]
            tunnel: w452 -> [w708]
            tunnel: w451 -> [w707]
            i -> [w705]
            w719 = TRUE ("averaging")
            w768 = TRUE ("init/cont (init:F)")
            n273 = Dequeue Element(queue=w774, error in (no error)=w773) -> (queue out=w770:refnum<queue>, element=w710:waveform(dbl)[], error out=w769:errorcluster)  [unwired: 2 out]
            n274 = Index Array(array=w710) -> (element #1=w767:waveform(dbl), element #2=w766:waveform(dbl), element #3=w765:waveform(dbl), element #4=w764:waveform(dbl), element #5=w763:waveform(dbl), element #6=w762:waveform(dbl), element #7=w761:waveform(dbl), element #8=w760:waveform(dbl))  [unwired: 8 in]
            n275 = Unbundle By Name(w767) -> ("Y"=w759:dbl[])
            n276 = Unbundle By Name(w766) -> ("Y"=w758:dbl[])
            n277 = Unbundle By Name(w765) -> ("Y"=w757:dbl[])
            n278 = Unbundle By Name(w764) -> ("Y"=w756:dbl[])
            n279 = Unbundle By Name(w763) -> ("Y"=w755:dbl[])
            n280 = Unbundle By Name(w762) -> ("Y"=w754:dbl[])
            n281 = Unbundle By Name(w761) -> ("Y"=w753:dbl[])
            n282 = Unbundle By Name(w760) -> ("Y"=w752:dbl[])
            n283 = Multiply(x=w759, y=w709) -> (x*y=w734:dbl[])
            n284 = Multiply(x=w758, y=w709) -> (x*y=w733:dbl[])
            n285 = Multiply(x=w757, y=w709) -> (x*y=w732:dbl[])
            n286 = Multiply(x=w756, y=w709) -> (x*y=w731:dbl[])
            n287 = Multiply(x=w755, y=w709) -> (x*y=w730:dbl[])
            n288 = Multiply(x=w754, y=w709) -> (x*y=w729:dbl[])
            n289 = Multiply(x=w753, y=w709) -> (x*y=w728:dbl[])
            n290 = Multiply(x=w752, y=w709) -> (x*y=w727:dbl[])
            n291 = call-poly <vilib>:"Decimate (single shot).vi"("averaging"=w719, "decimating factor"=w708, "X"=w729) -> ("Decimated Array"=w722:dbl[])  [unwired: 7 in, 1 out]
            n292 = call-poly <vilib>:"Decimate (single shot).vi"("averaging"=w719, "decimating factor"=w708, "X"=w727) -> ("Decimated Array"=w720:dbl[])  [unwired: 7 in, 1 out]
            n293 = call-poly <vilib>:"Decimate (single shot).vi"("averaging"=w719, "decimating factor"=w708, "X"=w733) -> ("Decimated Array"=w726:dbl[])  [unwired: 7 in, 1 out]
            n294 = call-poly <vilib>:"Decimate (single shot).vi"("averaging"=w719, "decimating factor"=w708, "X"=w731) -> ("Decimated Array"=w724:dbl[])  [unwired: 7 in, 1 out]
            n295 = call-poly <vilib>:"Decimate (single shot).vi"("averaging"=w719, "decimating factor"=w708, "X"=w730) -> ("Decimated Array"=w723:dbl[])  [unwired: 7 in, 1 out]
            n296 = call-poly <vilib>:"Decimate (single shot).vi"("averaging"=w719, "decimating factor"=w708, "X"=w728) -> ("Decimated Array"=w721:dbl[])  [unwired: 7 in, 1 out]
            n297 = call-poly <vilib>:"Decimate (single shot).vi"("averaging"=w719, "decimating factor"=w708, "X"=w734) -> ("Decimated Array"=w735:dbl[])  [unwired: 7 in, 1 out]
            n298 = call-poly <vilib>:"Decimate (single shot).vi"("averaging"=w719, "decimating factor"=w708, "X"=w732) -> ("Decimated Array"=w725:dbl[])  [unwired: 7 in, 1 out]
            n299 = call-poly <vilib>:"FIR Filter.vi"("init/cont (init:F)"=w768, "FIR Coefficients"=w707, "X"=w735) -> ("Filtered X"=w751:dbl[])  [unwired: 1 in, 1 out]
            n300 = call-poly <vilib>:"FIR Filter.vi"("init/cont (init:F)"=w768, "FIR Coefficients"=w707, "X"=w726) -> ("Filtered X"=w750:dbl[])  [unwired: 1 in, 1 out]
            n301 = call-poly <vilib>:"FIR Filter.vi"("init/cont (init:F)"=w768, "FIR Coefficients"=w707, "X"=w725) -> ("Filtered X"=w749:dbl[])  [unwired: 1 in, 1 out]
            n302 = call-poly <vilib>:"FIR Filter.vi"("init/cont (init:F)"=w768, "FIR Coefficients"=w707, "X"=w724) -> ("Filtered X"=w748:dbl[])  [unwired: 1 in, 1 out]
            n303 = call-poly <vilib>:"FIR Filter.vi"("init/cont (init:F)"=w768, "FIR Coefficients"=w707, "X"=w723) -> ("Filtered X"=w747:dbl[])  [unwired: 1 in, 1 out]
            n304 = call-poly <vilib>:"FIR Filter.vi"("init/cont (init:F)"=w768, "FIR Coefficients"=w707, "X"=w722) -> ("Filtered X"=w746:dbl[])  [unwired: 1 in, 1 out]
            n305 = call-poly <vilib>:"FIR Filter.vi"("init/cont (init:F)"=w768, "FIR Coefficients"=w707, "X"=w721) -> ("Filtered X"=w745:dbl[])  [unwired: 1 in, 1 out]
            n306 = call-poly <vilib>:"FIR Filter.vi"("init/cont (init:F)"=w768, "FIR Coefficients"=w707, "X"=w720) -> ("Filtered X"=w744:dbl[])  [unwired: 1 in, 1 out]
            n307 = call "Envelope(SubVI).vi"("x"=w751) -> ("Y"=w743:dbl[])
            n308 = call "Envelope(SubVI).vi"("x"=w750) -> ("Y"=w742:dbl[])
            n309 = call "Envelope(SubVI).vi"("x"=w749) -> ("Y"=w741:dbl[])
            n310 = call "Envelope(SubVI).vi"("x"=w748) -> ("Y"=w740:dbl[])
            n311 = call "Envelope(SubVI).vi"("x"=w747) -> ("Y"=w739:dbl[])
            n312 = call "Envelope(SubVI).vi"("x"=w746) -> ("Y"=w738:dbl[])
            n313 = call "Envelope(SubVI).vi"("x"=w745) -> ("Y"=w737:dbl[])
            n314 = call "Envelope(SubVI).vi"("x"=w744) -> ("Y"=w736:dbl[])
            n315 = Square(x=w743) -> (x^2=w718:dbl[])
            n316 = Square(x=w742) -> (x^2=w717:dbl[])
            n317 = Square(x=w741) -> (x^2=w716:dbl[])
            n318 = Square(x=w740) -> (x^2=w715:dbl[])
            n319 = Square(x=w739) -> (x^2=w714:dbl[])
            n320 = Square(x=w738) -> (x^2=w713:dbl[])
            n321 = Square(x=w737) -> (x^2=w712:dbl[])
            n322 = Square(x=w736) -> (x^2=w711:dbl[])
            n323 = Build Array(w718, w717, w716, w715, w714, w713, w712, w711) -> (w706:dbl[][])
            n324 = Enqueue Element(queue=w772, element=w706, error in (no error)=w771) -> ()  [unwired: 1 in, 3 out]
            "숫자형 6" <- w705
          }
          n325 = Release Queue(queue=w465, error in (no error)=w464) -> ()  [unwired: 1 in, 3 out]
          n326 = Obtain Queue(name (unnamed)=w416, element data type=w414) -> (queue out=w463:refnum<queue>, error out=w462:errorcluster)  [unwired: 3 in, 1 out]
          n327 = Obtain Queue(name (unnamed)=w457, element data type=w456) -> (queue out=w461:refnum<queue>, error out=w460:errorcluster)  [unwired: 3 in, 1 out]
          n328 = for {
            N: w409 -> [_]
            tunnel: w461 -> [w704]
            tunnel: w460 -> [w703]
            tunnel: w463 -> [w702]
            tunnel: w462 -> [w701]
            tunnel: [w700] -> w459
            tunnel: [w699] -> w458
            tunnel: w453 -> [w639]
            tunnel: w452 -> [w638]
            tunnel: w450 -> [w637]
            i -> [w635]
            w649 = TRUE ("averaging")
            w698 = TRUE ("init/cont (init:F)")
            n329 = Dequeue Element(queue=w704, error in (no error)=w703) -> (queue out=w700:refnum<queue>, element=w640:waveform(dbl)[], error out=w699:errorcluster)  [unwired: 2 out]
            n330 = Index Array(array=w640) -> (element #1=w697:waveform(dbl), element #2=w696:waveform(dbl), element #3=w695:waveform(dbl), element #4=w694:waveform(dbl), element #5=w693:waveform(dbl), element #6=w692:waveform(dbl), element #7=w691:waveform(dbl), element #8=w690:waveform(dbl))  [unwired: 8 in]
            n331 = Unbundle By Name(w697) -> ("Y"=w689:dbl[])
            n332 = Unbundle By Name(w696) -> ("Y"=w688:dbl[])
            n333 = Unbundle By Name(w695) -> ("Y"=w687:dbl[])
            n334 = Unbundle By Name(w694) -> ("Y"=w686:dbl[])
            n335 = Unbundle By Name(w693) -> ("Y"=w685:dbl[])
            n336 = Unbundle By Name(w692) -> ("Y"=w684:dbl[])
            n337 = Unbundle By Name(w691) -> ("Y"=w683:dbl[])
            n338 = Unbundle By Name(w690) -> ("Y"=w682:dbl[])
            n339 = Multiply(x=w689, y=w639) -> (x*y=w664:dbl[])
            n340 = Multiply(x=w688, y=w639) -> (x*y=w663:dbl[])
            n341 = Multiply(x=w687, y=w639) -> (x*y=w662:dbl[])
            n342 = Multiply(x=w686, y=w639) -> (x*y=w661:dbl[])
            n343 = Multiply(x=w685, y=w639) -> (x*y=w660:dbl[])
            n344 = Multiply(x=w684, y=w639) -> (x*y=w659:dbl[])
            n345 = Multiply(x=w683, y=w639) -> (x*y=w658:dbl[])
            n346 = Multiply(x=w682, y=w639) -> (x*y=w657:dbl[])
            n347 = call-poly <vilib>:"Decimate (single shot).vi"("averaging"=w649, "decimating factor"=w638, "X"=w659) -> ("Decimated Array"=w652:dbl[])  [unwired: 7 in, 1 out]
            n348 = call-poly <vilib>:"Decimate (single shot).vi"("averaging"=w649, "decimating factor"=w638, "X"=w657) -> ("Decimated Array"=w650:dbl[])  [unwired: 7 in, 1 out]
            n349 = call-poly <vilib>:"Decimate (single shot).vi"("averaging"=w649, "decimating factor"=w638, "X"=w663) -> ("Decimated Array"=w656:dbl[])  [unwired: 7 in, 1 out]
            n350 = call-poly <vilib>:"Decimate (single shot).vi"("averaging"=w649, "decimating factor"=w638, "X"=w661) -> ("Decimated Array"=w654:dbl[])  [unwired: 7 in, 1 out]
            n351 = call-poly <vilib>:"Decimate (single shot).vi"("averaging"=w649, "decimating factor"=w638, "X"=w660) -> ("Decimated Array"=w653:dbl[])  [unwired: 7 in, 1 out]
            n352 = call-poly <vilib>:"Decimate (single shot).vi"("averaging"=w649, "decimating factor"=w638, "X"=w658) -> ("Decimated Array"=w651:dbl[])  [unwired: 7 in, 1 out]
            n353 = call-poly <vilib>:"Decimate (single shot).vi"("averaging"=w649, "decimating factor"=w638, "X"=w664) -> ("Decimated Array"=w665:dbl[])  [unwired: 7 in, 1 out]
            n354 = call-poly <vilib>:"Decimate (single shot).vi"("averaging"=w649, "decimating factor"=w638, "X"=w662) -> ("Decimated Array"=w655:dbl[])  [unwired: 7 in, 1 out]
            n355 = call-poly <vilib>:"FIR Filter.vi"("init/cont (init:F)"=w698, "FIR Coefficients"=w637, "X"=w665) -> ("Filtered X"=w681:dbl[])  [unwired: 1 in, 1 out]
            n356 = call-poly <vilib>:"FIR Filter.vi"("init/cont (init:F)"=w698, "FIR Coefficients"=w637, "X"=w656) -> ("Filtered X"=w680:dbl[])  [unwired: 1 in, 1 out]
            n357 = call-poly <vilib>:"FIR Filter.vi"("init/cont (init:F)"=w698, "FIR Coefficients"=w637, "X"=w655) -> ("Filtered X"=w679:dbl[])  [unwired: 1 in, 1 out]
            n358 = call-poly <vilib>:"FIR Filter.vi"("init/cont (init:F)"=w698, "FIR Coefficients"=w637, "X"=w654) -> ("Filtered X"=w678:dbl[])  [unwired: 1 in, 1 out]
            n359 = call-poly <vilib>:"FIR Filter.vi"("init/cont (init:F)"=w698, "FIR Coefficients"=w637, "X"=w653) -> ("Filtered X"=w677:dbl[])  [unwired: 1 in, 1 out]
            n360 = call-poly <vilib>:"FIR Filter.vi"("init/cont (init:F)"=w698, "FIR Coefficients"=w637, "X"=w652) -> ("Filtered X"=w676:dbl[])  [unwired: 1 in, 1 out]
            n361 = call-poly <vilib>:"FIR Filter.vi"("init/cont (init:F)"=w698, "FIR Coefficients"=w637, "X"=w651) -> ("Filtered X"=w675:dbl[])  [unwired: 1 in, 1 out]
            n362 = call-poly <vilib>:"FIR Filter.vi"("init/cont (init:F)"=w698, "FIR Coefficients"=w637, "X"=w650) -> ("Filtered X"=w674:dbl[])  [unwired: 1 in, 1 out]
            n363 = call "Envelope(SubVI).vi"("x"=w681) -> ("Y"=w673:dbl[])
            n364 = call "Envelope(SubVI).vi"("x"=w680) -> ("Y"=w672:dbl[])
            n365 = call "Envelope(SubVI).vi"("x"=w679) -> ("Y"=w671:dbl[])
            n366 = call "Envelope(SubVI).vi"("x"=w678) -> ("Y"=w670:dbl[])
            n367 = call "Envelope(SubVI).vi"("x"=w677) -> ("Y"=w669:dbl[])
            n368 = call "Envelope(SubVI).vi"("x"=w676) -> ("Y"=w668:dbl[])
            n369 = call "Envelope(SubVI).vi"("x"=w675) -> ("Y"=w667:dbl[])
            n370 = call "Envelope(SubVI).vi"("x"=w674) -> ("Y"=w666:dbl[])
            n371 = Square(x=w673) -> (x^2=w648:dbl[])
            n372 = Square(x=w672) -> (x^2=w647:dbl[])
            n373 = Square(x=w671) -> (x^2=w646:dbl[])
            n374 = Square(x=w670) -> (x^2=w645:dbl[])
            n375 = Square(x=w669) -> (x^2=w644:dbl[])
            n376 = Square(x=w668) -> (x^2=w643:dbl[])
            n377 = Square(x=w667) -> (x^2=w642:dbl[])
            n378 = Square(x=w666) -> (x^2=w641:dbl[])
            n379 = Build Array(w648, w647, w646, w645, w644, w643, w642, w641) -> (w636:dbl[][])
            n380 = Enqueue Element(queue=w702, element=w636, error in (no error)=w701) -> ()  [unwired: 1 in, 3 out]
            "숫자형 7" <- w635
          }
          n381 = Release Queue(queue=w459, error in (no error)=w458) -> ()  [unwired: 1 in, 3 out]
          n382 = Obtain Queue(name (unnamed)=w415, element data type=w414) -> (queue out=w420:refnum<queue>, error out=w419:errorcluster)  [unwired: 3 in, 1 out]
          n383 = Obtain Queue(name (unnamed)=w416, element data type=w414) -> (queue out=w418:refnum<queue>, error out=w417:errorcluster)  [unwired: 3 in, 1 out]
          n384 = for {
            N: w409 -> [_]
            tunnel: w420 -> [w634]
            tunnel: w419 -> [w633]
            tunnel: w418 -> [w632]
            tunnel: w417 -> [w631]
            tunnel: w411 -> [w629]
            tunnel: w410 -> [w593]
            tunnel: [w541] -> _
            tunnel: [w540] -> _
            tunnel: [w539] -> _
            tunnel: [w538] -> _
            tunnel: w412 -> [w537]
            shift-right: [w511] -> _
            shift-left: w413 -> [w527]
            shift-right: [w510] -> _
            shift-left: w413 -> [w526]
            shift-right: [w509] -> _
            shift-left: w413 -> [w525]
            shift-right: [w508] -> _
            shift-left: w413 -> [w524]
            shift-right: [w507] -> _
            shift-left: w413 -> [w523]
            shift-right: [w506] -> _
            shift-left: w413 -> [w522]
            shift-right: [w505] -> _
            shift-left: w413 -> [w521]
            shift-right: [w504] -> _
            shift-left: w413 -> [w520]
            i -> [w536]
            w618 = enum32{"Peaks", "Valleys"}."Valleys" ("peaks/valleys")
            w619 = enum32{"Peaks", "Valleys"}."Peaks" ("peaks/valleys")
            w617 = 5 ("width")
            w628 = TRUE ("init/cont (init:F)")
            n385 = Dequeue Element(queue=w634, error in (no error)=w633) -> (queue out=w541:refnum<queue>, element=w575:dbl[][], error out=w540:errorcluster)  [unwired: 2 out]
            n386 = Dequeue Element(queue=w632, error in (no error)=w631) -> (queue out=w539:refnum<queue>, element=w574:dbl[][], error out=w538:errorcluster)  [unwired: 2 out]
            n387 = Subtract(x=w575, y=w574) -> (x-y=w630:dbl[][])
            n388 = Index Array(array=w630) -> (element #1=w616:dbl[], element #2=w615:dbl[], element #3=w614:dbl[], element #4=w613:dbl[], element #5=w612:dbl[], element #6=w611:dbl[], element #7=w610:dbl[], element #8=w578:dbl[])  [unwired: 16 in]
            n389 = call-poly <vilib>:"FIR Filter.vi"("init/cont (init:F)"=w628, "FIR Coefficients"=w629, "X"=w616) -> ("Filtered X"=w627:dbl[])  [unwired: 1 in, 1 out]
            n390 = call-poly <vilib>:"FIR Filter.vi"("init/cont (init:F)"=w628, "FIR Coefficients"=w629, "X"=w615) -> ("Filtered X"=w626:dbl[])  [unwired: 1 in, 1 out]
            n391 = call-poly <vilib>:"FIR Filter.vi"("init/cont (init:F)"=w628, "FIR Coefficients"=w629, "X"=w614) -> ("Filtered X"=w625:dbl[])  [unwired: 1 in, 1 out]
            n392 = call-poly <vilib>:"FIR Filter.vi"("init/cont (init:F)"=w628, "FIR Coefficients"=w629, "X"=w613) -> ("Filtered X"=w624:dbl[])  [unwired: 1 in, 1 out]
            n393 = call-poly <vilib>:"FIR Filter.vi"("init/cont (init:F)"=w628, "FIR Coefficients"=w629, "X"=w612) -> ("Filtered X"=w623:dbl[])  [unwired: 1 in, 1 out]
            n394 = call-poly <vilib>:"FIR Filter.vi"("init/cont (init:F)"=w628, "FIR Coefficients"=w629, "X"=w611) -> ("Filtered X"=w622:dbl[])  [unwired: 1 in, 1 out]
            n395 = call-poly <vilib>:"FIR Filter.vi"("init/cont (init:F)"=w628, "FIR Coefficients"=w629, "X"=w610) -> ("Filtered X"=w621:dbl[])  [unwired: 1 in, 1 out]
            n396 = call-poly <vilib>:"FIR Filter.vi"("init/cont (init:F)"=w628, "FIR Coefficients"=w629, "X"=w578) -> ("Filtered X"=w620:dbl[])  [unwired: 1 in, 1 out]
            n397 = Array Max & Min(array=w627) -> (max value=w609:dbl, min value=w608:dbl)  [unwired: 2 out]
            n398 = Array Max & Min(array=w626) -> (max value=w607:dbl, min value=w606:dbl)  [unwired: 2 out]
            n399 = Array Max & Min(array=w625) -> (max value=w605:dbl, min value=w604:dbl)  [unwired: 2 out]
            n400 = Array Max & Min(array=w624) -> (max value=w603:dbl, min value=w602:dbl)  [unwired: 2 out]
            n401 = Array Max & Min(array=w623) -> (max value=w601:dbl, min value=w600:dbl)  [unwired: 2 out]
            n402 = Array Max & Min(array=w622) -> (max value=w599:dbl, min value=w598:dbl)  [unwired: 2 out]
            n403 = Array Max & Min(array=w621) -> (max value=w597:dbl, min value=w596:dbl)  [unwired: 2 out]
            n404 = Array Max & Min(array=w620) -> (max value=w595:dbl, min value=w594:dbl)  [unwired: 2 out]
            n405 = call "ThresholdEstimation(SubVI).vi"("Margin"=w593, "최소값"=w606, "최대값"=w607) -> ("N.Th"=w580:dbl, "P.Th"=w591:dbl)
            n406 = call "ThresholdEstimation(SubVI).vi"("Margin"=w593, "최소값"=w604, "최대값"=w605) -> ("N.Th"=w581:dbl, "P.Th"=w590:dbl)
            n407 = call "ThresholdEstimation(SubVI).vi"("Margin"=w593, "최소값"=w602, "최대값"=w603) -> ("N.Th"=w582:dbl, "P.Th"=w589:dbl)
            n408 = call "ThresholdEstimation(SubVI).vi"("Margin"=w593, "최소값"=w600, "최대값"=w601) -> ("N.Th"=w583:dbl, "P.Th"=w588:dbl)
            n409 = call "ThresholdEstimation(SubVI).vi"("Margin"=w593, "최소값"=w608, "최대값"=w609) -> ("N.Th"=w579:dbl, "P.Th"=w592:dbl)
            n410 = call "ThresholdEstimation(SubVI).vi"("Margin"=w593, "최소값"=w598, "최대값"=w599) -> ("N.Th"=w584:dbl, "P.Th"=w587:dbl)
            n411 = call "ThresholdEstimation(SubVI).vi"("Margin"=w593, "최소값"=w596, "최대값"=w597) -> ("N.Th"=w585:dbl, "P.Th"=w586:dbl)
            n412 = call "ThresholdEstimation(SubVI).vi"("Margin"=w593, "최소값"=w594, "최대값"=w595) -> ("N.Th"=w577:dbl, "P.Th"=w576:dbl)
            n413 = call <vilib>:"Peak Detector.vi"("peaks/valleys"=w619, "width"=w617, "threshold"=w592, "X"=w616) -> ("Locations"=w550:dbl[], "# found"=w566:i32)  [unwired: 3 in, 3 out]
            n414 = call <vilib>:"Peak Detector.vi"("peaks/valleys"=w619, "width"=w617, "threshold"=w591, "X"=w615) -> ("Locations"=w551:dbl[], "# found"=w567:i32)  [unwired: 3 in, 3 out]
            n415 = call <vilib>:"Peak Detector.vi"("peaks/valleys"=w619, "width"=w617, "threshold"=w590, "X"=w614) -> ("Locations"=w552:dbl[], "# found"=w568:i32)  [unwired: 3 in, 3 out]
            n416 = call <vilib>:"Peak Detector.vi"("peaks/valleys"=w619, "width"=w617, "threshold"=w589, "X"=w613) -> ("Locations"=w553:dbl[], "# found"=w569:i32)  [unwired: 3 in, 3 out]
            n417 = call <vilib>:"Peak Detector.vi"("peaks/valleys"=w619, "width"=w617, "threshold"=w588, "X"=w612) -> ("Locations"=w554:dbl[], "# found"=w570:i32)  [unwired: 3 in, 3 out]
            n418 = call <vilib>:"Peak Detector.vi"("peaks/valleys"=w619, "width"=w617, "threshold"=w587, "X"=w611) -> ("Locations"=w555:dbl[], "# found"=w571:i32)  [unwired: 3 in, 3 out]
            n419 = call <vilib>:"Peak Detector.vi"("peaks/valleys"=w619, "width"=w617, "threshold"=w586, "X"=w610) -> ("Locations"=w556:dbl[], "# found"=w572:i32)  [unwired: 3 in, 3 out]
            n420 = call <vilib>:"Peak Detector.vi"("peaks/valleys"=w619, "width"=w617, "threshold"=w576, "X"=w578) -> ("Locations"=w557:dbl[], "# found"=w573:i32)  [unwired: 3 in, 3 out]
            n421 = call <vilib>:"Peak Detector.vi"("peaks/valleys"=w618, "width"=w617, "threshold"=w579, "X"=w616) -> ("Locations"=w549:dbl[], "# found"=w565:i32)  [unwired: 3 in, 3 out]
            n422 = call <vilib>:"Peak Detector.vi"("peaks/valleys"=w618, "width"=w617, "threshold"=w580, "X"=w615) -> ("Locations"=w548:dbl[], "# found"=w564:i32)  [unwired: 3 in, 3 out]
            n423 = call <vilib>:"Peak Detector.vi"("peaks/valleys"=w618, "width"=w617, "threshold"=w581, "X"=w614) -> ("Locations"=w547:dbl[], "# found"=w563:i32)  [unwired: 3 in, 3 out]
            n424 = call <vilib>:"Peak Detector.vi"("peaks/valleys"=w618, "width"=w617, "threshold"=w582, "X"=w613) -> ("Locations"=w546:dbl[], "# found"=w562:i32)  [unwired: 3 in, 3 out]
            n425 = call <vilib>:"Peak Detector.vi"("peaks/valleys"=w618, "width"=w617, "threshold"=w583, "X"=w612) -> ("Locations"=w545:dbl[], "# found"=w561:i32)  [unwired: 3 in, 3 out]
            n426 = call <vilib>:"Peak Detector.vi"("peaks/valleys"=w618, "width"=w617, "threshold"=w584, "X"=w611) -> ("Locations"=w544:dbl[], "# found"=w560:i32)  [unwired: 3 in, 3 out]
            n427 = call <vilib>:"Peak Detector.vi"("peaks/valleys"=w618, "width"=w617, "threshold"=w585, "X"=w610) -> ("Locations"=w543:dbl[], "# found"=w559:i32)  [unwired: 3 in, 3 out]
            n428 = call <vilib>:"Peak Detector.vi"("peaks/valleys"=w618, "width"=w617, "threshold"=w577, "X"=w578) -> ("Locations"=w542:dbl[], "# found"=w558:i32)  [unwired: 3 in, 3 out]
            n429 = call "Decision(SubVI).vi"("L_ind0"=w566, "L_ind1"=w565, "Peak_ind0"=w550, "Peak_ind1"=w549) -> ("L_sum"=w519:i32, "Bits"=w535:dbl[])  [unwired: 2 in]
            n430 = call "Decision(SubVI).vi"("L_ind0"=w567, "L_ind1"=w564, "Peak_ind0"=w551, "Peak_ind1"=w548) -> ("L_sum"=w518:i32, "Bits"=w534:dbl[])  [unwired: 2 in]
            n431 = call "Decision(SubVI).vi"("L_ind0"=w568, "L_ind1"=w563, "Peak_ind0"=w552, "Peak_ind1"=w547) -> ("L_sum"=w517:i32, "Bits"=w533:dbl[])  [unwired: 2 in]
            n432 = call "Decision(SubVI).vi"("L_ind0"=w569, "L_ind1"=w562, "Peak_ind0"=w553, "Peak_ind1"=w546) -> ("L_sum"=w516:i32, "Bits"=w532:dbl[])  [unwired: 2 in]
            n433 = call "Decision(SubVI).vi"("L_ind0"=w570, "L_ind1"=w561, "Peak_ind0"=w554, "Peak_ind1"=w545) -> ("L_sum"=w515:i32, "Bits"=w531:dbl[])  [unwired: 2 in]
            n434 = call "Decision(SubVI).vi"("L_ind0"=w571, "L_ind1"=w560, "Peak_ind0"=w555, "Peak_ind1"=w544) -> ("L_sum"=w514:i32, "Bits"=w530:dbl[])  [unwired: 2 in]
            n435 = call "Decision(SubVI).vi"("L_ind0"=w572, "L_ind1"=w559, "Peak_ind0"=w556, "Peak_ind1"=w543) -> ("L_sum"=w513:i32, "Bits"=w529:dbl[])  [unwired: 2 in]
            n436 = call "Decision(SubVI).vi"("L_ind0"=w573, "L_ind1"=w558, "Peak_ind0"=w557, "Peak_ind1"=w542) -> ("L_sum"=w512:i32, "Bits"=w528:dbl[])  [unwired: 2 in]
            n437 = call "DataBuffer(SubVI).vi"("Bits"=w535, "Buffer"=w527) -> ("Data"=w511:dbl[])  [unwired: 2 in]
            n438 = call "DataBuffer(SubVI).vi"("Bits"=w534, "Buffer"=w526) -> ("Data"=w510:dbl[])  [unwired: 2 in]
            n439 = call "DataBuffer(SubVI).vi"("Bits"=w533, "Buffer"=w525) -> ("Data"=w509:dbl[])  [unwired: 2 in]
            n440 = call "DataBuffer(SubVI).vi"("Bits"=w532, "Buffer"=w524) -> ("Data"=w508:dbl[])  [unwired: 2 in]
            n441 = call "DataBuffer(SubVI).vi"("Bits"=w531, "Buffer"=w523) -> ("Data"=w507:dbl[])  [unwired: 2 in]
            n442 = call "DataBuffer(SubVI).vi"("Bits"=w530, "Buffer"=w522) -> ("Data"=w506:dbl[])  [unwired: 2 in]
            n443 = call "DataBuffer(SubVI).vi"("Bits"=w529, "Buffer"=w521) -> ("Data"=w505:dbl[])  [unwired: 2 in]
            n444 = call "DataBuffer(SubVI).vi"("Bits"=w528, "Buffer"=w520) -> ("Data"=w504:dbl[])  [unwired: 2 in]
            n445 = call "CodeDetection(SubVI).vi"("Code"=w537, "Buff"=w511, "L_sum"=w519) -> ()  [unwired: 1 out]
            n446 = call "CodeDetection(SubVI).vi"("Code"=w537, "Buff"=w510, "L_sum"=w518) -> ()  [unwired: 1 out]
            n447 = call "CodeDetection(SubVI).vi"("Code"=w537, "Buff"=w509, "L_sum"=w517) -> ()  [unwired: 1 out]
            n448 = call "CodeDetection(SubVI).vi"("Code"=w537, "Buff"=w508, "L_sum"=w516) -> ()  [unwired: 1 out]
            n449 = call "CodeDetection(SubVI).vi"("Code"=w537, "Buff"=w507, "L_sum"=w515) -> ()  [unwired: 1 out]
            n450 = call "CodeDetection(SubVI).vi"("Code"=w537, "Buff"=w506, "L_sum"=w514) -> ()  [unwired: 1 out]
            n451 = call "CodeDetection(SubVI).vi"("Code"=w537, "Buff"=w505, "L_sum"=w513) -> ()  [unwired: 1 out]
            n452 = call "CodeDetection(SubVI).vi"("Code"=w537, "Buff"=w504, "L_sum"=w512) -> ()  [unwired: 1 out]
            "숫자형 8" <- w536
          }
        }
      }
    }
  }
